vi "Build Timing Command.vi"(8 "error in":errorcluster, 11 "3300 in":refnum<class "3300.lvclass">) -> (0 "error out":errorcluster, 2 "resulting string":string, 3 "3300 out":refnum<class "3300.lvclass">)   [LabVIEW 2019, in "3300.lvlib" / "3300.lvclass"]
uses:
  Library/3300.lvclass
  C:/Users/Public/Documents/Development/builds/Instruments/Electronic Load.lvlibp/Library/Electronic Load.lvclass
  builds/Instruments/Electronic Load.lvlibp/Accessors/Trigger/Read Pulse Sample Interval.vi
  builds/Instruments/Electronic Load.lvlibp/Accessors/Trigger/Read Pulse Data Points.vi
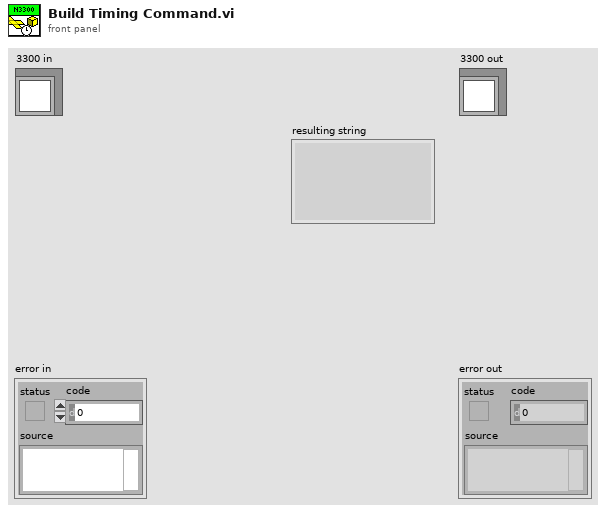
[diagram p1: front panel]
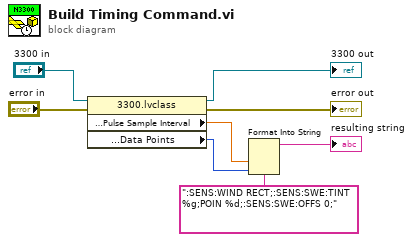
[diagram p0: block diagram]
diagram:
  n1 = property class="3300.lvclass"(reference="3300 in", error in="error in") -> (reference out=→"3300 out":refnum<class "3300.lvclass">, error out=→"error out":errorcluster, "Accessors:Settings:Pulse:Pulse Sample Interval"=w4:dbl, "Accessors:Settings:Pulse:Data Points"=w3:i32)
  n2 = Format Into String(format string=":SENS:WIND RECT;:SENS:SWE:TINT %g;POIN %d;:SENS:SWE:OFFS 0;", w4, w3) -> (resulting string=→"resulting string":string)  [unwired: 2 in, 1 out]
